vi "Add new Guardian.vi"(8 "error in (no error)":errorcluster, 9 "Guardian Properties":T1, 10 "ID":string, 11 "Guardian List in":refnum<class "Guardian List.lvclass">) -> (0 "error out":errorcluster, 3 "Guardian List out":refnum<class "Guardian List.lvclass">)   [LabVIEW 2026, in "TALOS.lvlib" / "Classes.lvlib" / "Guardian List.lvclass"]
uses:
  Guardian List.lvclass
  Guardian Properties.ctl
  Guardian List.lvclass/Guardian List.ctl
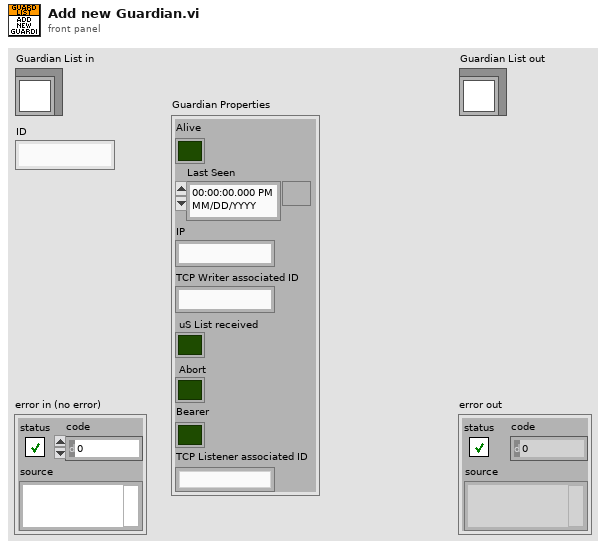
[diagram p1: front panel]
types:
  T1 = typedef "TALOS.lvlib/Classes.lvlib/Guardian List.lvclass/Guardian Properties.ctl" = cluster{"Alive":bool, "Last Seen":timestamp, "IP":string, "TCP Writer associated ID":string, "uS List received":bool, "Abort":bool, "Bearer":bool, "TCP Listener associated ID":string}
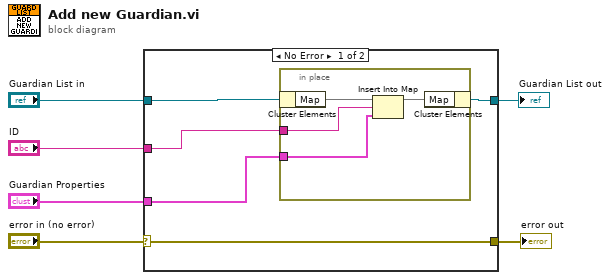
[diagram p0: block diagram]
diagram:
  n1 = case shown="No Error" "error in (no error)" {
    selector: "error in (no error)" -> [w9 w17]
    tunnel: [w9 w17] -> w5
    tunnel: [w10 w16] -> w3
    tunnel: "Guardian List in" -> [w11 w16]
    tunnel: "ID" -> [w8 _]
    tunnel: "Guardian Properties" -> [w7 _]
    frame No Error {
      n2 = in-place "In Place Element Structure" {
        in-place-border: w8 -> [w13]
        in-place-border: w7 -> [w12]
        n3 = in-place-cluster #1(w11) -> ("Map"=w15:map{string, T1})
        n4 = Insert Into Map(map in=w15, key=w13, value=w12) -> (map out=w14:map{string, T1})  [unwired: 2 out]
        n5 = in-place-cluster #1("Map"=w14) -> (w10:refnum<class "Guardian List.lvclass">)
      }
    }
    frame Error {
    }
  }
  "error out" <- w5
  "Guardian List out" <- w3
